vi "WaitForTCPResponse.vi"(2 "Action":string, 3 "Module Slot":string) -> (0 "Received Data":string, 1 "Ready":bool)   [LabVIEW 2016]
uses:
  GlobalControlVariables.vi
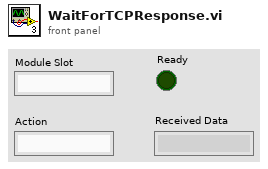
[diagram p1: front panel]
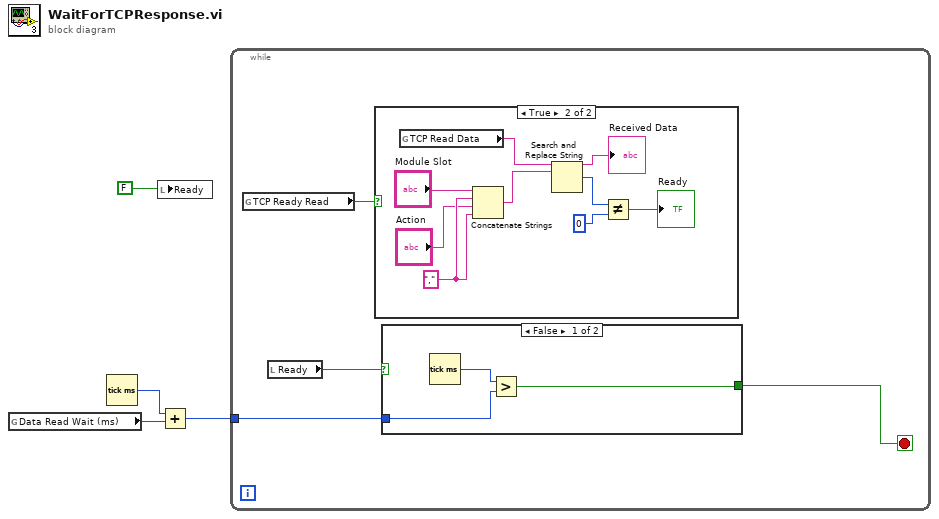
[diagram p0: block diagram]
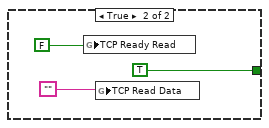
[diagram p2: hidden frame]
diagram:
  n1 = global read "GlobalControlVariables.vi" "Data Read Wait (ms)"() -> (w2:u32)
  n2 = Tick Count (ms)() -> (millisecond timer value=w3:u32)
  n3 = local write "Ready"(FALSE) -> ()
  n4 = Add(x=w3, y=w2) -> (x+y=w1:u32)
  n5 = while {
    tunnel: w1 -> [w6]
    stop <- w5 stop-if-true
    n6 = global read "GlobalControlVariables.vi" "TCP Ready Read"() -> (w8:bool)
    n7 = local read "Ready"() -> (w7:bool)
    n8 = case shown="True" w8 {
      frame False {
      }
      frame True {
        w21 = ","
        n9 = global read "GlobalControlVariables.vi" "TCP Read Data"() -> (w16:string)
        n10 = Concatenate Strings("Module Slot", w21, "Action", w21) -> (w15:string)
        n11 = Search and Replace String(input string=w16, search string=w15) -> (result string=→"Received Data":string, number of replacements=w18:i32)  [unwired: 6 in, 2 out]
        n12 = Not Equal?(x=w18, y=u32 0) -> (x != y?=→"Ready":bool)
      }
    }
    n13 = case shown="False" w7 {
      tunnel: [w9 TRUE] -> w5
      tunnel: w6 -> [w10 _]
      frame False {
        n14 = Tick Count (ms)() -> (millisecond timer value=w11:u32)
        n15 = Greater?(x=w11, y=w10) -> (0:w9:bool)
      }
      frame True {
        n16 = global write "GlobalControlVariables.vi" "TCP Ready Read"(FALSE) -> ()
        n17 = global write "GlobalControlVariables.vi" "TCP Read Data"("") -> ()
      }
    }
  }
